vi "MoistureSensorReset.vi"(0 "GEA2 Reference In":refnum<k24>, 11 "Error In":errorcluster) -> (4 "GEA2 Reference Out":refnum<k24>, 6 "Pass/Fail?":bool, 8 "Report Text":string, 15 "Error Out":errorcluster)   [LabVIEW 2019]
uses:
  D:/Common/LabVIEW GEA2 Toolkit/source/GEA3 DLL Source/GeaCommunication.dll
  Common/LabVIEW GEA2 Toolkit/source/GEA3 DLL Source/GeaCommunication.dll
  Common/LabVIEW GEA2 Toolkit/GEA3/type defs/Source_Destination.ctl
  Common/LabVIEW GEA2 Toolkit/GEA3/type defs/ERD Write Data In.ctl
  Common/LabVIEW GEA2 Toolkit/GEA3/type defs/Data Type.ctl
  Common/LabVIEW GEA2 Toolkit/GEA3/type defs/ERD Read Data In.ctl
  Common/LabVIEW GEA2 Toolkit/GEA3/library/GEA2_Toolkit.lvlib
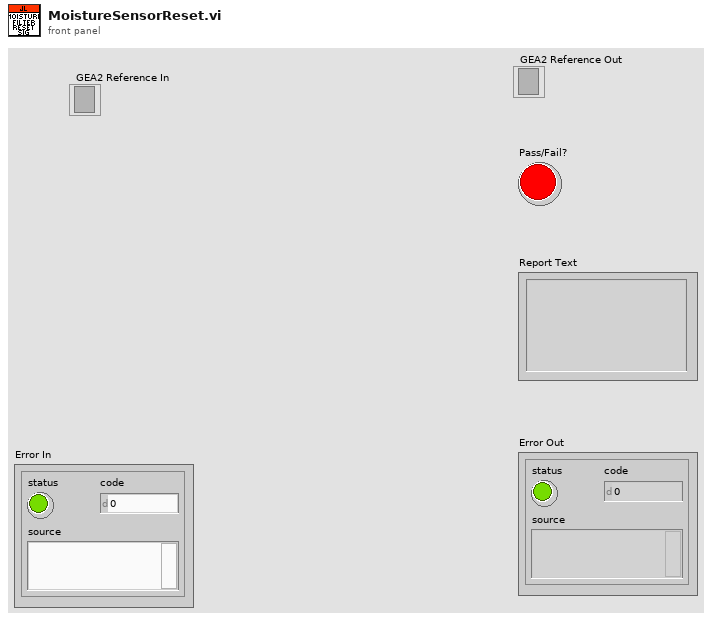
[diagram p1: front panel]
types:
  T1 = typedef "ERD Read Data In.ctl" = cluster{"ERD Number":u16, "Data Type":enum16{"string", "boolean", "uint8_t", "uint16_t", "uint32_t", "uint64_t", "int8_t", "int16_t", "int32_t", "int64_t"}}
  T2 = typedef "ERD Write Data In.ctl" = cluster{"ERD Number":u16, "Data Type":T3, "Data":string}
  T3 = typedef "Data Type.ctl" = enum16{"string", "boolean", "uint8_t", "uint16_t", "uint32_t", "uint64_t", "int8_t", "int16_t", "int32_t", "int64_t"}
  T4 = typedef "Source_Destination.ctl" = cluster{"Source":u8, "Destination":u8}
  T5 = typedef "ERD Read Data Out.ctl" = cluster{"ERD Number":u16, "Data":string}
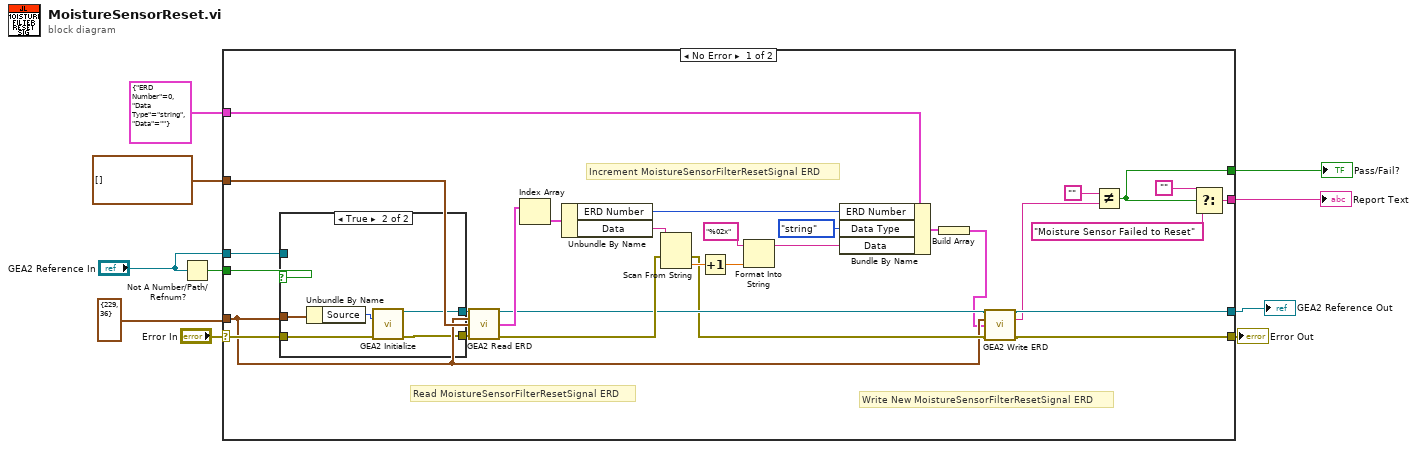
[diagram p0: block diagram]
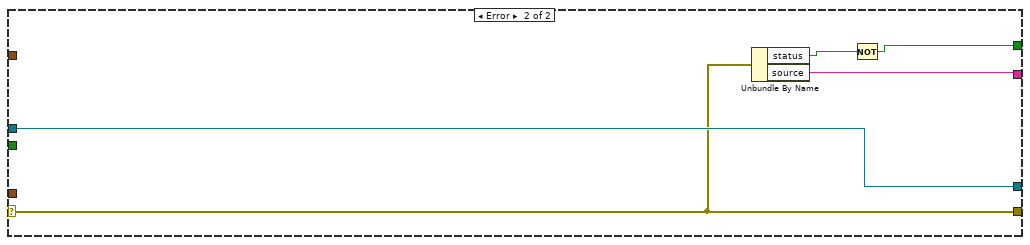
[diagram p3: hidden frame]
diagram:
  n1 = Not A Number/Path/Refnum?(number/path/refnum="GEA2 Reference In") -> (NaN/Path/Refnum?=w10:bool)
  n2 = case shown="No Error" "Error In" {
    selector: "Error In" -> [w27 w51]
    tunnel: [w17 w52] -> w2
    tunnel: w10 -> [w29 _]
    tunnel: "GEA2 Reference In" -> [w28 w52]
    tunnel: T4 {"Source"=229, "Destination"=36} ("GEA Inputs") -> [w12 _]
    tunnel: T2 {"ERD Number"=0, "Data Type"=enum."string", "Data"=""} ("ERD Write Data In") -> [w25 _]
    tunnel: T1[] [] ("Read ERD List") -> [w24 _]
    tunnel: [w14 w51] -> w5
    tunnel: [w21 w48] -> w3
    tunnel: [w20 w50] -> w4
    frame No Error {
      # "Write New MoistureSensorFilterResetSignal ERD"
      # "Increment MoistureSensorFilterResetSignal ERD"
      # "Read MoistureSensorFilterResetSignal ERD"
      n3 = case shown="True" w29 {
        tunnel: w12 -> [_ w47]
        tunnel: [w42 w45] -> w31
        tunnel: w28 -> [w42 _]
        tunnel: w27 -> [w41 w44]
        tunnel: [w41 w43] -> w26
        frame False {
        }
        frame True {
          n4 = Unbundle By Name(w47) -> ("Source"=w46:u8)
          n5 = call "GEA2 Initialize.vi"("Source Address"=w46, "error in"=w44) -> ("GEA2 Reference Out"=w45:refnum<k24>, "error out"=w43:errorcluster)  [unwired: 11 in, 1 out]
        }
      }
      n6 = call "GEA2 Read ERD.vi"("GEA2 Reference In"=w31, "GEA Inputs"=w12, "Read ERD List"=w24, "Error In"=w26) -> ("GEA2 Reference Out"=w16:refnum<k24>, "ERD Data Out"=w40:T5[], "Error Out"=w18:errorcluster)  [unwired: 8 in, 1 out]
      n7 = Index Array(array=w40) -> (element=w39:T5)  [unwired: 1 in]
      n8 = Unbundle By Name(w39) -> ("ERD Number"=w38:u16, "Data"=w36:string)
      n9 = Scan From String(input string=w36, error in=w18) -> (error out=w15:errorcluster, output 1=w35:dbl)  [unwired: 3 in, 2 out]
      n10 = Increment(x=w35) -> (x+1=w34:dbl)
      n11 = Format Into String(format string="%02x", w34) -> (resulting string=w33:string)  [unwired: 2 in, 1 out]
      n12 = Bundle By Name(cluster=w25, "ERD Number"=w38, "Data Type"=Data_Type."string", "Data"=w33) -> (w32:T2)
      n13 = Build Array(w32) -> (w11:T2[])
      n14 = call "GEA2 Write ERD.vi"("GEA2 Reference In"=w16, "GEA Inputs"=w12, "Write ERD List"=w11, "Error In"=w15) -> ("GEA2 Reference Out"=w17:refnum<k24>, "Raw Data Out"=w13:string, "Error Out"=w14:errorcluster)  [unwired: 9 in]
      n15 = Not Equal?(x="", y=w13) -> (x != y?=w21:bool)
      n16 = Select(t="", s=w21, f="Moisture Sensor Failed to Reset") -> (s? t:f=w20:string)
    }
    frame Error {
      n17 = Unbundle By Name(w51) -> ("status"=w49:bool, "source"=w50:string)
      n18 = Not(x=w49) -> (.not. x?=w48:bool)
    }
  }
  "GEA2 Reference Out" <- w2
  "Error Out" <- w5
  "Report Text" <- w4
  "Pass/Fail?" <- w3
